vi "DAQ Main.vi"() -> ()   [LabVIEW 2017]
uses:
  Controls/RT- Queue States.ctl
  Code/TCP/TCP Engine/Controls/TCP - Driver Control State.ctl
  Code/TCP/TCP Host/Controls/Control - Testscreen.ctl
  Test cycle Execution/Control/Test Cycle Execution_States.ctl
  SubVIs/SubVI - Global.vi
  <vilib>/FPGAPlugInAG/cRIO-9034/niLvFpga_Open_cRIO-9034.vi
  <vilib>/rvi/interface/common/dynamic/niFpgaDynamicAddResources.vi
  <vilib>/Utility/error.llb/Error Cluster From Error Code.vi
  <vilib>/rvi/errors/niLvFpgaAdjustHostInterfaceError.vi
  <vilib>/Utility/file.llb/Write Delimited Spreadsheet (string).vi
  <vilib>/rvi/interface/nirviOpenFPGA/nirviOpenFPGA.xnode
  FPGA Bitfiles/TataSteel_FPGATarget_FPGA-Main_ZcEZVGyWzKA.lvbitx
  <vilib>/rvi/interface/nirviReadWriteControl/nirviReadWriteControl.xnode
  <vilib>/rvi/interface/nirviMethod/nirviMethod.xnode
  <vilib>/FPGAPlugInAG/Dynamic/niLvFpga_ReadFifo_Dynamic.vi
  <vilib>/rvi/errors/niLvFpgaMergeErrorWithErrorCode.vi
  NiFpgaLv.dll
  <vilib>/rvi/interface/Simulation/niFpgaSimulationCallBeginRW.vi
panel:
  out "SW Heartbeat":bool
  out "File Transfer":bool
  out "Datalog Interval":dbl
  out "Boolean":bool
  out "DII":bool[](array[boolean])
  out "variant":variant
  in  "Auto Trigger Data":bool
  in  "Mod1 Data":i32=2
  out "DI Data":i32[](array[numeric])
  out "Faults":bool[](array[boolean])
  out "Elapsed Time":dbl
  out "Live DI Data":u32[](array[numeric])
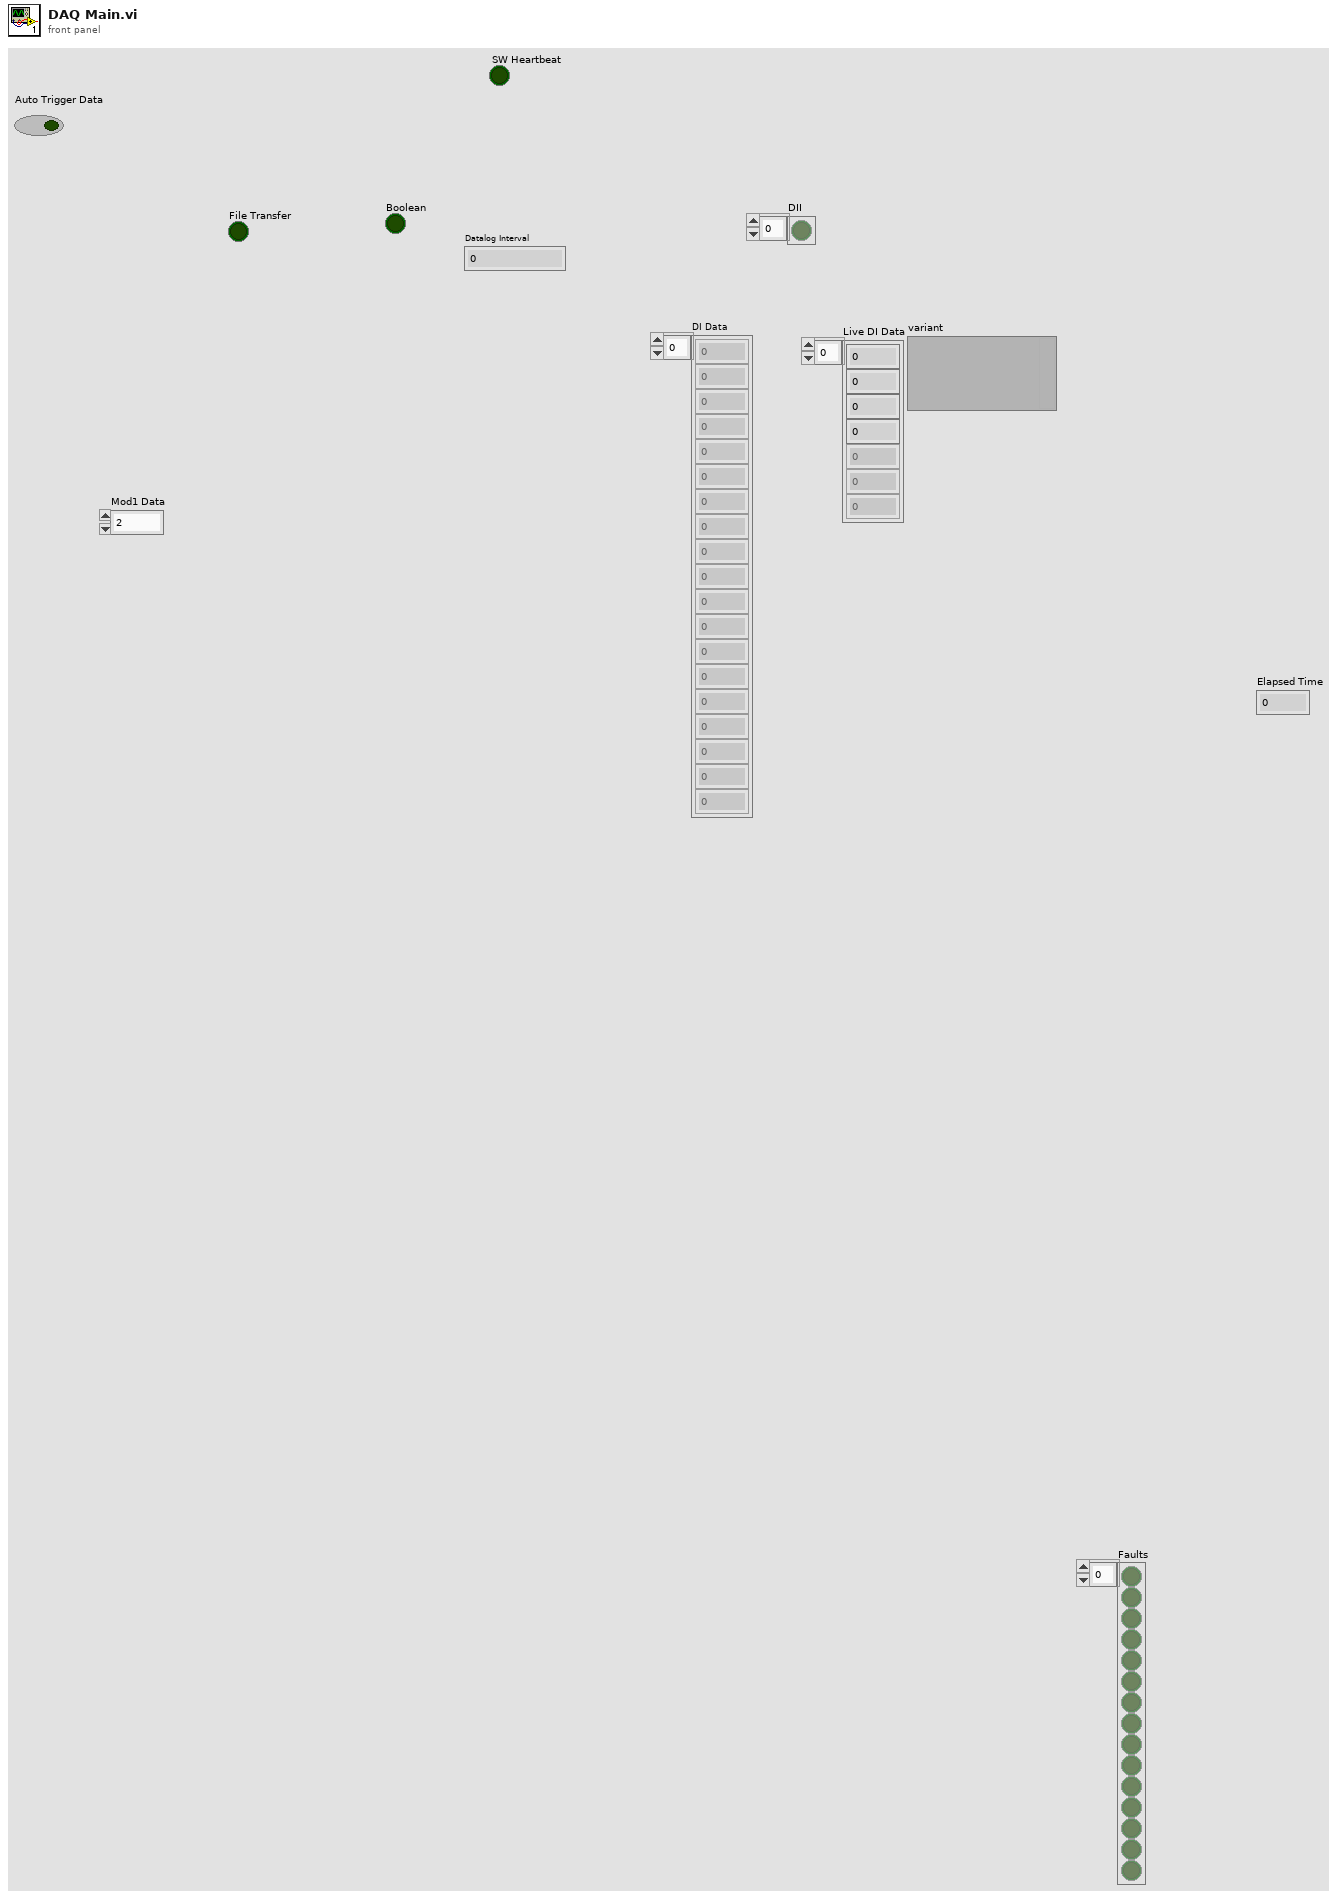
[diagram p1: front panel]
types:
  T1 = typedef "RT- Queue States.ctl" = enum16{"Initialize", "Enqueue", "Enqueue Priority", "Dequeue", "Flush", "Destroy"}
  T2 = typedef "Control - Testscreen.ctl" = enum16{"No Event", "Init", "Load Settings", "Save Setting", "Save Test Info", "Get Report", "Download Files", "Test Running", "Update Test Results", "Machine Unhealthy", "Autotest Started", "Test Aborted", "Sequence Complete", "Update Sensor Data", "Log File Available", "Machine Mode", "Aux Logging Started", "Aux File Saved", "Get PID Values", "View Report", "Exit", "Wait", "Abort", "Copy Log File", "Generate Alarm", "Send Test Details"}
  T3 = typedef "TCP - Driver Control State.ctl" = enum16{"Test Settings", "Send Test Details", "Boolean Commands", "Test Results"}
  T4 = typedef "Test Cycle Execution_States.ctl" = enum16{"Download Config Files", "Test Started", "Test Running", "Update Sensor Data", "Test Complete"}
  T5 = cluster{"Histogram Data":i16[], "Sensor Data":i16[], "File Path":path}
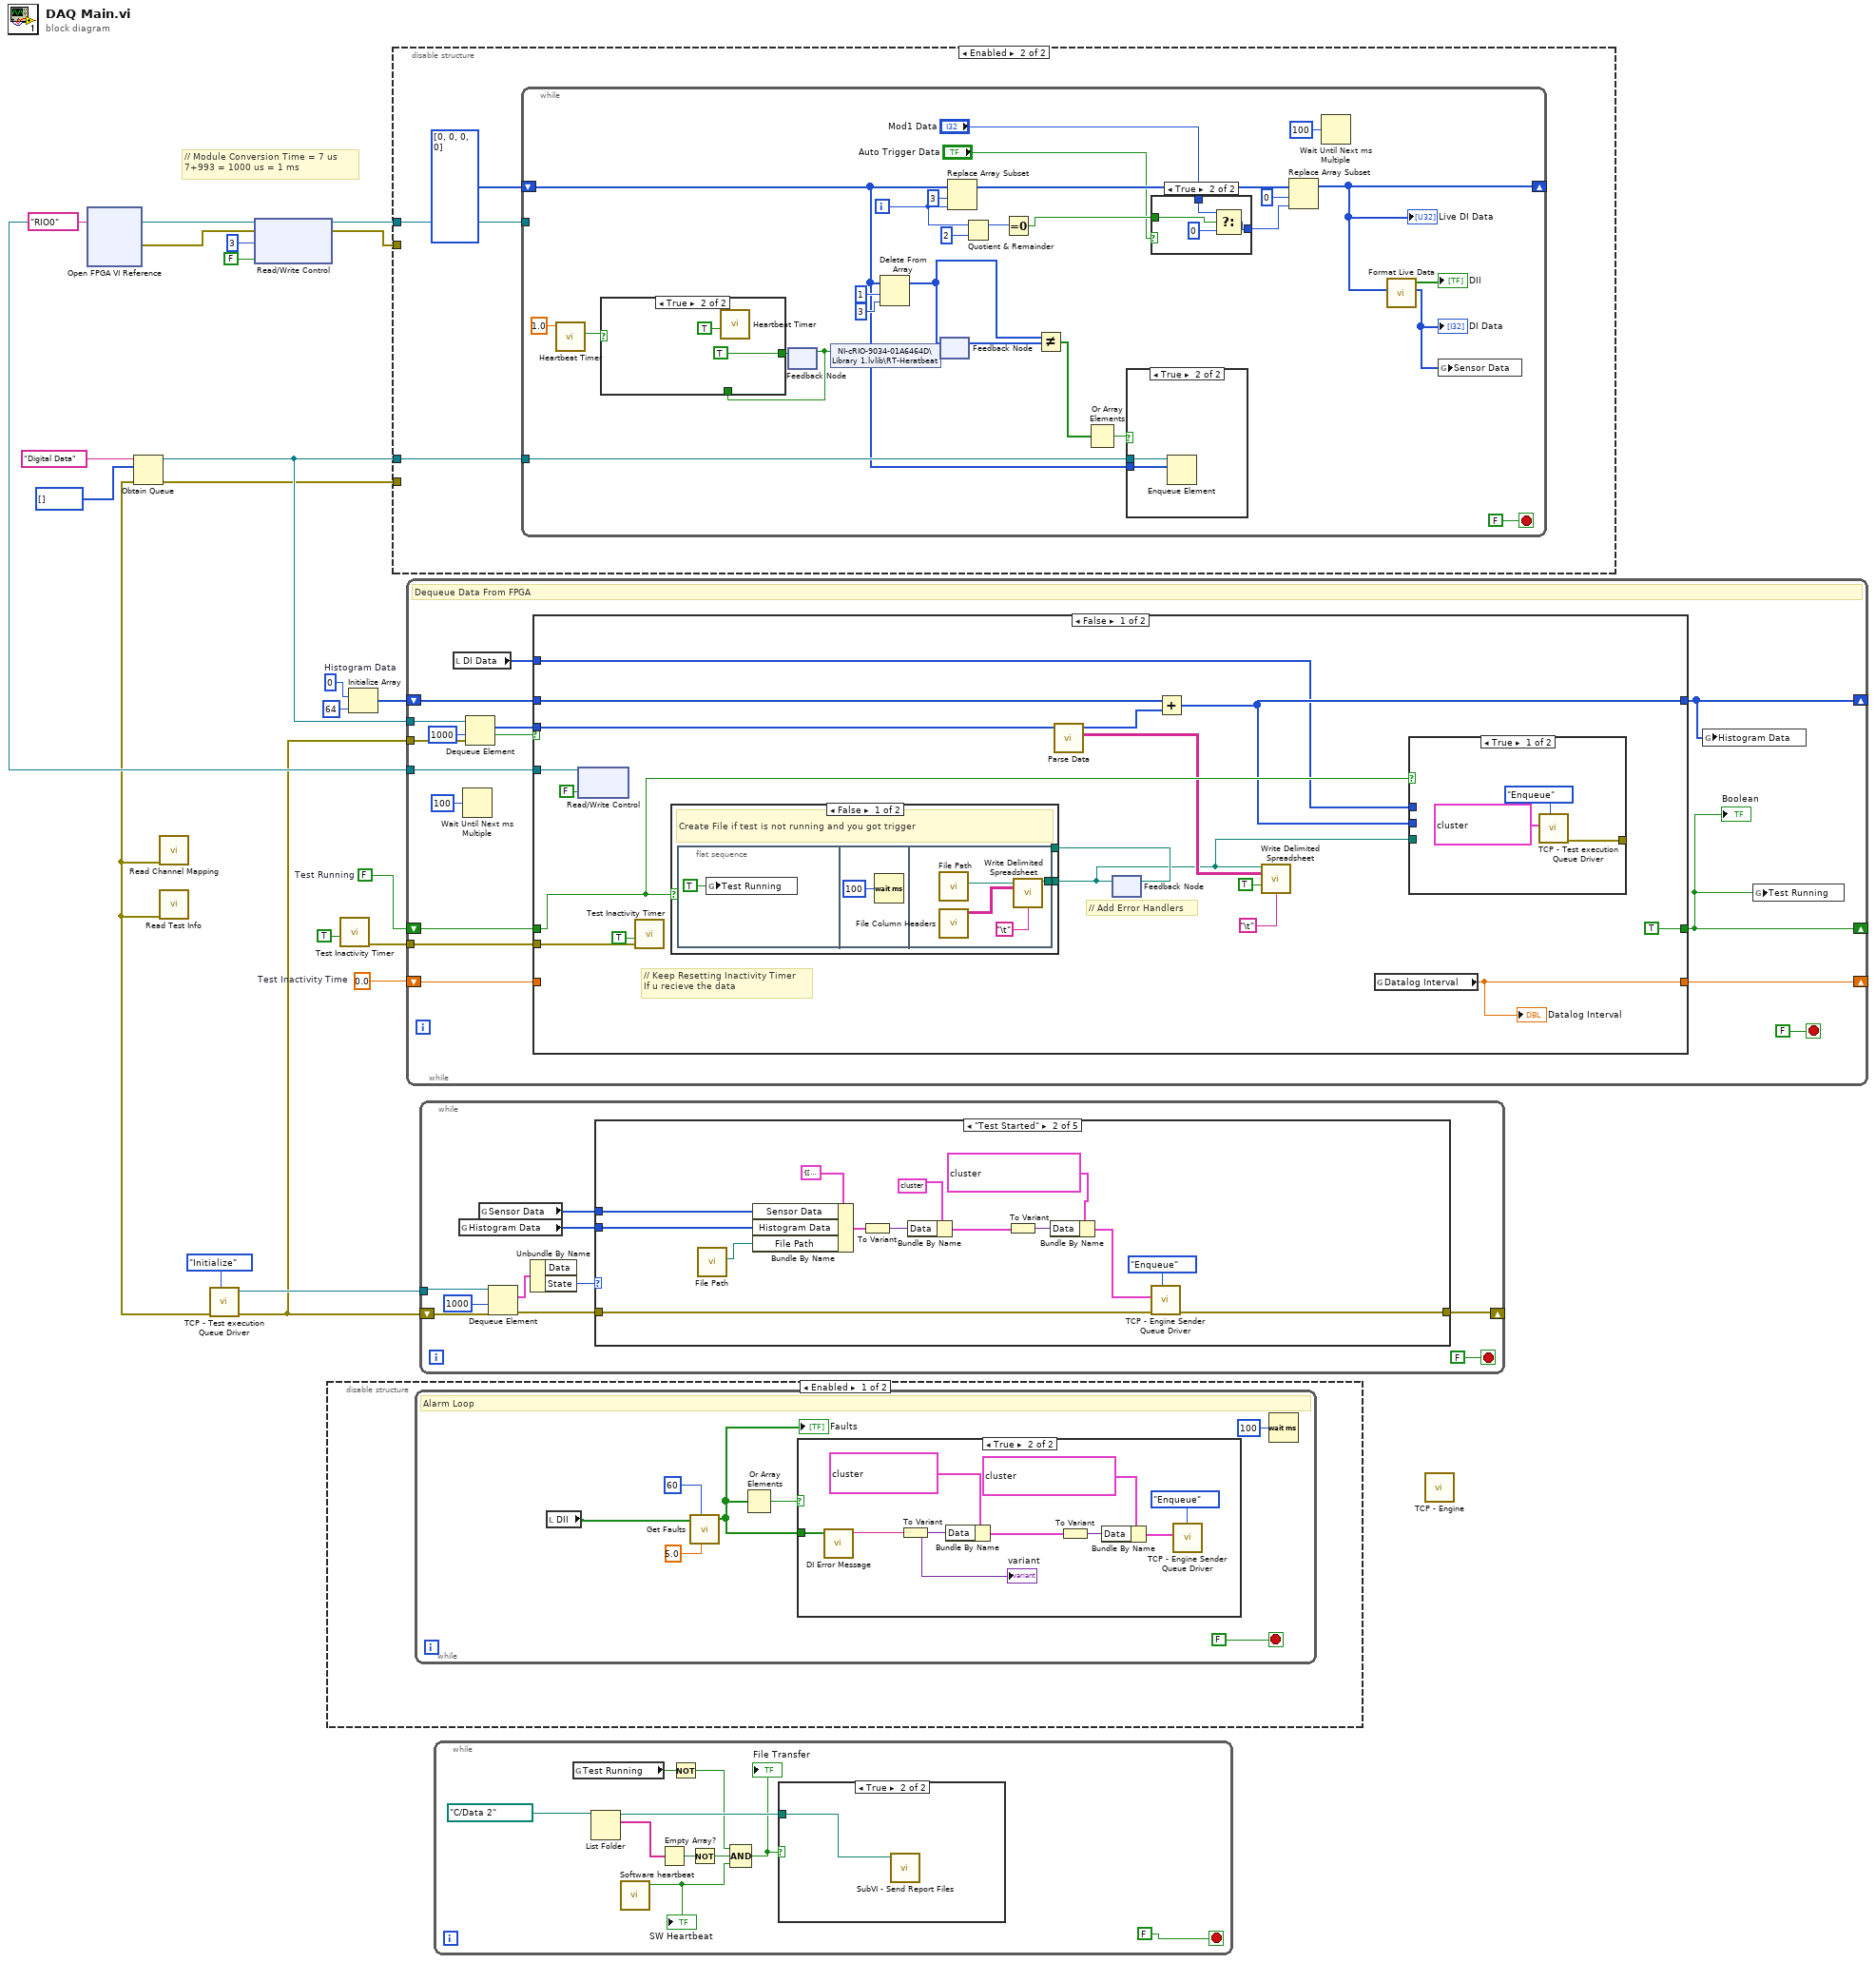
[diagram p0: block diagram]
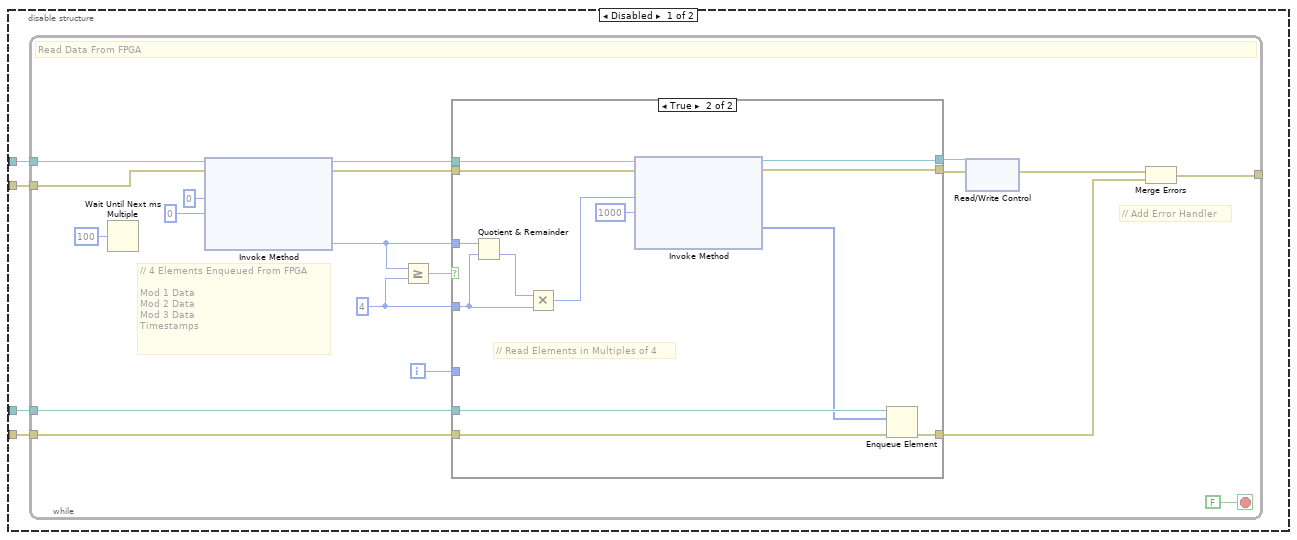
[diagram p5: hidden frame]
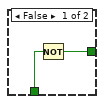
[diagram p7: hidden frame]
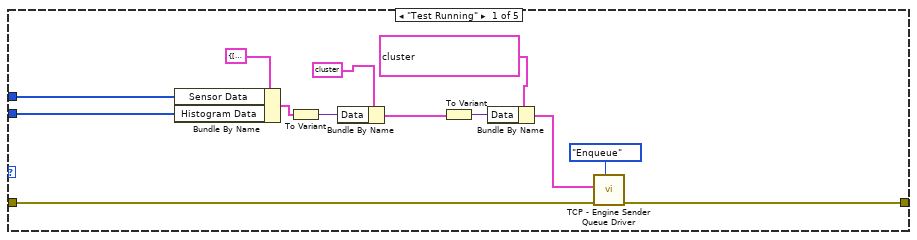
[diagram p10: hidden frame]
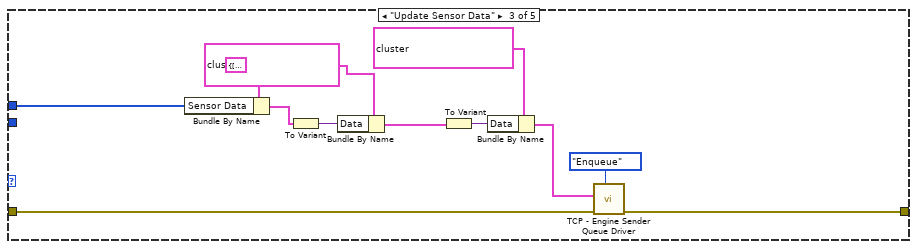
[diagram p11: hidden frame]
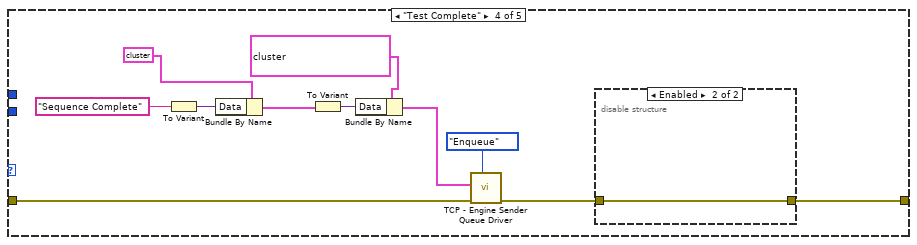
[diagram p12: hidden frame]
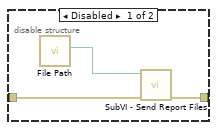
[diagram p13: hidden frame]
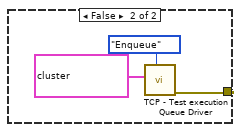
[diagram p15: hidden frame]
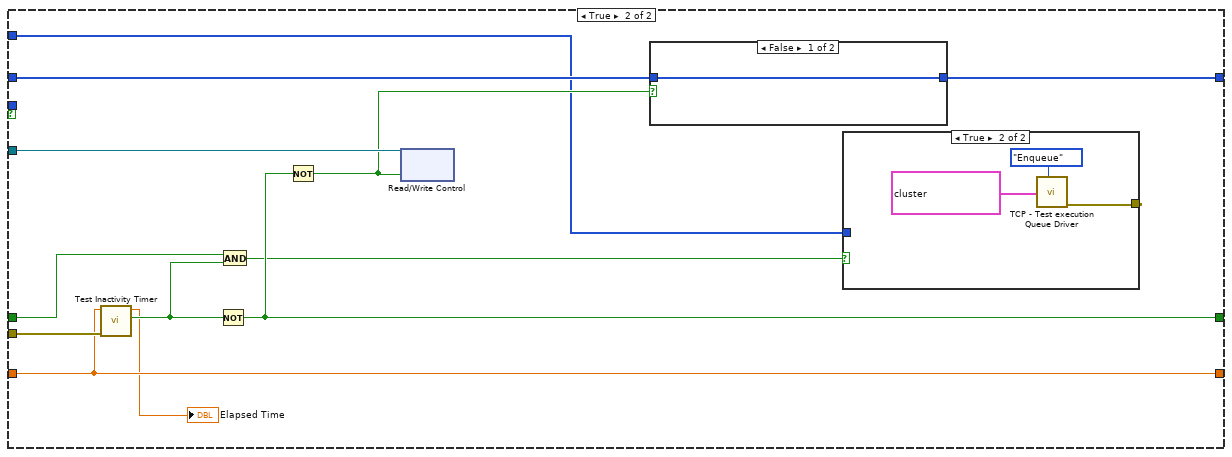
[diagram p17: hidden frame]
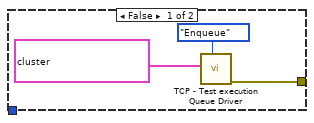
[diagram p18: hidden frame]
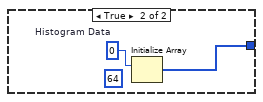
[diagram p19: hidden frame]
diagram:
  w4 = i16 0  # Histogram Data
  w15 = 0.0  # Test Inactivity Time
  w16 = FALSE  # Test Running
  # "// Module Conversion Time = 7 us\n7+993 = 1000 us = 1 ms"
  n1 = xnode "Open FPGA VI Reference"("resource name"=tag "RIO0") -> ("FPGA VI Reference Out"=w8:refnum<k20>, "error out"=w10:errorcluster)  [unwired: 1 in]
  n2 = Obtain Queue(name (unnamed)="Digital Data", element data type=u64[] [] ("Data")) -> (queue out=w19:refnum<queue>, error out=w1:errorcluster)  [unwired: 3 in, 1 out]
  n3 = call "Read Channel Mapping.vi"("error in (no error)"=w1) -> ()  [unwired: 11 in]
  n4 = call "Read Test Info.vi"("error in (no error)"=w1) -> ()  [unwired: 11 in]
  n5 = call "TCP - Test execution Queue Driver.vi"("Cases"=RT-_Queue_States."Initialize", "error in (no error)"=w1) -> ("error out"=w5:errorcluster, "queue out"=w6:refnum<queue>)  [unwired: 7 in, 1 out]
  n6 = xnode "Read/Write Control"("FPGA VI Reference In"=w8, "error in"=w10, "Wait(uSec)"=u32 3, "Manual Log"=FALSE) -> ("FPGA VI Reference Out"=w12:refnum<k20>, "error out"=w9:errorcluster)
  n7 = disable-structure shown="Enabled" {
    frame Enabled {
      n8 = while {
        stop <- FALSE ("stop") stop-if-true
        # "Alarm Loop"
        n9 = local read "DII"() -> (w22:bool[])
        n10 = call "Get Faults.vi"("Timer(Sec)"=5.0, "No of Inputs"=60, "Inputs"=w22) -> ("Faults"=w23:bool[])  [unwired: 8 in]
        "Faults" <- w23
        n11 = Or Array Elements(Boolean array=w23) -> (logical OR=w24:bool)
        n12 = case shown="True" w24 {
          tunnel: w23 -> [_ w33]
          frame False {
          }
          frame True {
            n13 = call "DI Error Message.vi"("Faults"=w33) -> ("Error Message"=w29:string)  [unwired: 10 in]
            n14 = To Variant(anything=w29) -> (Variant=w36:variant)
            "variant" <- w36
            n15 = Bundle By Name(cluster=cluster{"Data":variant, "Enum":T2} {"Data"=variant, "Enum"=enum."Generate Alarm"} ("Element In"), "Data"=w36) -> (w32:cluster{"Data":variant, "Enum":T2})
            n16 = To Variant(anything=w32) -> (Variant=w37:variant)
            n17 = Bundle By Name(cluster=cluster{"Data":variant, "State":T3} {"Data"=variant, "State"=enum."Boolean Commands"} ("Element In"), "Data"=w37) -> (w35:cluster{"Data":variant, "State":T3})
            n18 = call "TCP - Engine Sender Queue Driver.vi"("Cases"=RT-_Queue_States."Enqueue", "Element In"=w35) -> ()  [unwired: 7 in, 3 out]
          }
        }
        n19 = Wait (ms)(milliseconds to wait=u32 100) -> ()  [unwired: 1 out]
      }
    }
    frame Disabled {
    }
  }
  n20 = call "Test Inactivity Timer.vi"("Reset"=TRUE) -> ("error out"=w17:errorcluster)  [unwired: 8 in, 2 out]
  n21 = Initialize Array(w4, 64 ("dimension size")) -> (w3:i16[])
  n22 = disable-structure shown="Enabled" {
    disable-tunnel: w19 -> [w41 w78]
    disable-tunnel: w12 -> [w40 w79]
    disable-tunnel: w9 -> [w39 _]
    disable-tunnel: w1 -> [w38 _]
    frame Disabled {
      n23 = while {
        tunnel: w40 -> [w45]
        tunnel: w39 -> [w55]
        tunnel: w41 -> [w52]
        tunnel: w38 -> [w51]
        tunnel: [w49] -> _
        i -> [w46]
        stop <- FALSE stop-if-true
        w57 = u32 4 ("y")
        # "// Add Error Handler"
        # "// 4 Elements Enqueued From FPGA\n\nMod 1 Data\nMod 2 Data\nMod 3 Data\nTimestamps"
        # "Read Data From FPGA"
        n24 = Wait Until Next ms Multiple(millisecond multiple=u32 100) -> ()  [unwired: 1 out]
        n25 = xnode "Invoke Method"("FPGA VI Reference In"=w45, "error in"=w55, "Number of Elements"=u32 0, "Timeout (ms)"=0) -> ("FPGA VI Reference Out"=w54:refnum<k20>, "error out"=w53:errorcluster, "Elements Remaining"=w58:u32)  [unwired: 1 out]
        n26 = Greater Or Equal?(x=w58, y=w57) -> (x >= y?=w56:bool)
        n27 = case shown="True" w56 {
          tunnel: w58 -> [_ w76]
          tunnel: w57 -> [_ w74]
          tunnel: w54 -> [w61 w73]
          tunnel: w53 -> [w63 w72]
          tunnel: w52 -> [_ w69]
          tunnel: w51 -> [w62 w68]
          tunnel: [w63 w66] -> w43
          tunnel: [w62 w65] -> w50
          tunnel: w46 -> [_ _]
          tunnel: [w61 w64] -> w44
          frame False {
          }
          frame True {
            # "// Read Elements in Multiples of 4"
            n28 = Quotient & Remainder(x=w76, y=w74) -> (floor(x/y)=w75:u32)  [unwired: 1 out]
            n29 = Multiply(x=w75, y=w74) -> (x*y=w71:u32)
            n30 = xnode "Invoke Method"("FPGA VI Reference In"=w73, "error in"=w72, "Number of Elements"=w71, "Timeout (ms)"=1000) -> ("FPGA VI Reference Out"=w64:refnum<k20>, "error out"=w66:errorcluster, "Data"=w67:u64[])  [unwired: 1 out]
            n31 = Enqueue Element(queue=w69, element=w67, error in (no error)=w68) -> (error out=w65:errorcluster)  [unwired: 1 in, 2 out]
          }
        }
        n32 = xnode "Read/Write Control"("FPGA VI Reference In"=w44, "error in"=w43) -> ("error out"=w42:errorcluster)  [unwired: 2 out]
        n33 = Merge Errors(w42, w50) -> (w49:errorcluster)
      }
    }
    frame Enabled {
      n34 = while {
        tunnel: w79 -> [_]
        tunnel: w78 -> [w106]
        shift-right: [w92] -> _
        shift-left: u32[] [0, 0, 0, 0] ("Simulation") -> [w89]
        i -> [w98]
        stop <- FALSE stop-if-true
        n35 = call "Heartbeat Timer.vi"("Target Time"=1.0) -> ("Time Elapsed"=w83:bool)  [unwired: 8 in, 2 out]
        n36 = feedback #1() -> (w80:bool)  [unwired: 1 in]
        n37 = case shown="True" w83 {
          tunnel: [w107 TRUE] -> w81
          tunnel: w80 -> [w108 _]
          frame False {
            n38 = Not(x=w108) -> (.not. x?=w107:bool)
          }
          frame True {
            n39 = call "Heartbeat Timer.vi"("Reset"=TRUE) -> ()  [unwired: 8 in, 3 out]
          }
        }
        n40 = feedback-in #1(w81) -> ()
        n41 = shared-variable "NI-cRIO-9034-01A6464D\\Library 1.lvlib\\RT-Heratbeat"(w80) -> ()  [unwired: 1 in, 1 out]
        n42 = Delete From Array(array=w89, length=1, index=3) -> (array with subset deleted=w88:u32[])  [unwired: 1 out]
        n43 = feedback-in #2(w88) -> ()
        n44 = feedback #2() -> (w104:u32[])  [unwired: 1 in]
        n45 = Replace Array Subset(array=w89, new element=w98, index=3) -> (w99:u32[])
        n46 = Quotient & Remainder(x=w98, y=2) -> (x-y*floor(x/y)=w96:i32)  [unwired: 1 out]
        n47 = Equal To 0?(x=w96) -> (x = 0?=w87:bool)
        n48 = Not Equal?(x=w88, y=w104) -> (x != y?=w103:bool[])
        n49 = Or Array Elements(Boolean array=w103) -> (logical OR=w102:bool)
        n50 = case shown="True" w102 {
          tunnel: w106 -> [_ w117]
          tunnel: w89 -> [_ w116]
          frame False {
          }
          frame True {
            n51 = Enqueue Element(queue=w117, element=w116) -> ()  [unwired: 2 in, 3 out]
          }
        }
        n52 = case shown="True" "Auto Trigger Data" {
          tunnel: "Mod1 Data" -> [w111 w115]
          tunnel: [w111 w113] -> w94
          tunnel: w87 -> [_ w112]
          frame False {
          }
          frame True {
            n53 = Select(t=w115, s=w112, f=0) -> (s? t:f=w113:i32)
          }
        }
        n54 = Replace Array Subset(array=w99, new element=w94, index=0) -> (w92:u32[])
        "Live DI Data" <- w92
        n55 = Wait Until Next ms Multiple(millisecond multiple=u32 100) -> ()  [unwired: 1 out]
        n56 = call "Format Live Data.vi"("Live DI Data"=w92) -> ("Array"=w105:i16[], "DII"=→"DII":bool[])  [unwired: 9 in]
        "DI Data" <- w105
        n57 = global write "SubVI - Global.vi" "Sensor Data"(w105) -> ()
      }
    }
  }
  n58 = while {
    tunnel: w19 -> [w133]
    tunnel: w5 -> [w132]
    tunnel: w17 -> [w127]
    shift-right: [w118] -> _
    shift-left: w16 -> [w126]
    shift-right: [w124] -> _
    shift-left: w15 -> [w125]
    tunnel: w8 -> [w122]
    shift-right: [w119] -> _
    shift-left: w3 -> [w121]
    stop <- FALSE stop-if-true
    # "Dequeue Data From FPGA"
    n59 = local read "DI Data"() -> (w120:i32[])
    n60 = Wait Until Next ms Multiple(millisecond multiple=u32 100) -> ()  [unwired: 1 out]
    n61 = Dequeue Element(queue=w133, timeout in ms (-1)=1000, error in (no error)=w132) -> (element=w131:u64[], timed out?=w128:bool)  [unwired: 2 out]
    n62 = case shown="False" w128 {
      tunnel: w131 -> [w150 _]
      tunnel: w127 -> [w148 w176]
      tunnel: w126 -> [w144 w167]
      tunnel: [TRUE w173] -> w118
      tunnel: w125 -> [_ w175]
      tunnel: [w135 w175] -> w124
      tunnel: w122 -> [w141 w174]
      tunnel: w121 -> [w143 w171]
      tunnel: [w142 w170] -> w119
      tunnel: w120 -> [w136 w165]
      frame False {
        # "// Add Error Handlers"
        # "// Keep Resetting Inactivity Timer\nIf u recieve the data"
        n63 = xnode "Read/Write Control"("FPGA VI Reference In"=w141, "Reset"=FALSE) -> ()  [unwired: 1 in, 2 out]
        n64 = call "Test Inactivity Timer.vi"("error in (no error)"=w148, "Reset"=TRUE) -> ()  [unwired: 7 in, 3 out]
        n65 = call "Parse Data.vi"("Data In"=w150) -> ("Values to Log"=w139:string[][], "Histogram Data"=w138:i16[])  [unwired: 9 in]
        n66 = feedback #3() -> (w145:path)  [unwired: 1 in]
        n67 = case shown="False" w144 {
          tunnel: [w157 w164] -> w137
          tunnel: w145 -> [_ w164]
          frame False {
            # "Create File if test is not running and you got trigger"
            n68 = flat-sequence {
              tunnel: [w162] -> w157
              frame #0 {
                n69 = global write "SubVI - Global.vi" "Test Running"(TRUE ("Test Running")) -> ()
              }
              frame #1 {
                n70 = Wait (ms)(milliseconds to wait=u32 100) -> ()  [unwired: 1 out]
              }
              frame #2 {
                n71 = call "File Path.vi"() -> ("File Path"=w161:path)  [unwired: 11 in]
                n72 = call "File Column Headers.vi"() -> ("Column Header"=w163:string[][])  [unwired: 11 in]
                n73 = call-poly <vilib>:"Write Delimited Spreadsheet.vi"("file path (dialog if empty)"=w161, "2D data"=w163, "delimiter (\\t)"="\t") -> ("new file path (Not A Path if cancelled)"=w162:path)  [unwired: 11 in, 1 out]
              }
            }
          }
          frame True {
          }
        }
        n74 = feedback-in #3(w137) -> ()
        n75 = Add(x=w143, y=w138) -> (x+y=w142:i16[])
        n76 = call-poly <vilib>:"Write Delimited Spreadsheet.vi"("file path (dialog if empty)"=w137, "2D data"=w139, "append to file? (new file:F)"=TRUE, "delimiter (\\t)"="\t") -> ()  [unwired: 10 in, 2 out]
        n77 = global read "SubVI - Global.vi" "Datalog Interval"() -> (w135:dbl)
        "Datalog Interval" <- w135
        n78 = case shown="True" w144 {
          tunnel: w136 -> [_ _]
          tunnel: w142 -> [_ _]
          tunnel: [w152 w155] -> _
          tunnel: w137 -> [_ _]
          frame True {
            n79 = call "TCP - Test execution Queue Driver.vi"("Cases"=RT-_Queue_States."Enqueue", "Element In"=cluster{"Data":variant, "State":T4} {"Data"=variant, "State"=enum."Test Running"}) -> ("error out"=w152:errorcluster)  [unwired: 7 in, 2 out]
          }
          frame False {
            n80 = call "TCP - Test execution Queue Driver.vi"("Cases"=RT-_Queue_States."Enqueue", "Element In"=cluster{"Data":variant, "State":T4} {"Data"=variant, "State"=enum."Test Started"}) -> ("error out"=w155:errorcluster)  [unwired: 7 in, 2 out]
          }
        }
      }
      frame True {
        n81 = call "Test Inactivity Timer.vi"("error in (no error)"=w176, "Target Time"=w175) -> ("Time Elapsed"=w169:bool, "Elapsed Time"=→"Elapsed Time":dbl)  [unwired: 7 in, 1 out]
        n82 = Not(x=w169) -> (.not. x?=w173:bool)
        n83 = And(x=w167, y=w169) -> (x .and. y?=w168:bool)
        n84 = Not(x=w173) -> (.not. x?=w172:bool)
        n85 = xnode "Read/Write Control"("FPGA VI Reference In"=w174, "Reset"=w172) -> ()  [unwired: 1 in, 2 out]
        n86 = case shown="False" w172 {
          tunnel: w171 -> [w183 _]
          tunnel: [w183 w184] -> w170
          frame False {
          }
          frame True {
            (unwired) 64 ("dimension size")
            w185 = i16 0  # Histogram Data
            n87 = Initialize Array(w185) -> (w184:i16[])  [unwired: 1 in]
          }
        }
        n88 = case shown="True" w168 {
          tunnel: w165 -> [_ _]
          tunnel: [w179 w182] -> _
          frame False {
            n89 = call "TCP - Test execution Queue Driver.vi"("Cases"=RT-_Queue_States."Enqueue", "Element In"=cluster{"Data":variant, "State":T4} {"Data"=variant, "State"=enum."Update Sensor Data"}) -> ("error out"=w179:errorcluster)  [unwired: 7 in, 2 out]
          }
          frame True {
            n90 = call "TCP - Test execution Queue Driver.vi"("Cases"=RT-_Queue_States."Enqueue", "Element In"=cluster{"Data":variant, "State":T4} {"Data"=variant, "State"=enum."Test Complete"}) -> ("error out"=w182:errorcluster)  [unwired: 7 in, 2 out]
          }
        }
      }
    }
    "Boolean" <- w118
    n91 = global write "SubVI - Global.vi" "Histogram Data"(w119) -> ()
    n92 = global write "SubVI - Global.vi" "Test Running"(w118) -> ()
  }
  n93 = while {
    shift-right: [w192] -> _
    shift-left: w5 -> [w193]
    tunnel: w6 -> [w194]
    stop <- FALSE stop-if-true
    n94 = global read "SubVI - Global.vi" "Histogram Data"() -> (w188:i32[])
    n95 = global read "SubVI - Global.vi" "Sensor Data"() -> (w187:i32[])
    n96 = Dequeue Element(queue=w194, timeout in ms (-1)=1000, error in (no error)=w193) -> (element=w190:cluster{"Data":variant, "State":T4}, error out=w191:errorcluster)  [unwired: 2 out]
    n97 = Unbundle By Name(w190) -> ("State"=w189:T4)  [unwired: 1 out]
    n98 = case shown="\"Test Started\"" w189 {
      tunnel: [w199 w213 w226 w238 w250] -> w192
      tunnel: w191 -> [w200 w214 w227 w241 w250]
      tunnel: w188 -> [w202 w216 _ _ _]
      tunnel: w187 -> [w201 w215 w228 _ _]
      frame "Test Running" {
        n99 = Bundle By Name(cluster=T5 {"Histogram Data"=[], "Sensor Data"=[], "File Path"=path ""}, "Sensor Data"=w201, "Histogram Data"=w202) -> (w208:T5)
        n100 = To Variant(anything=w208) -> (Variant=w206:variant)
        n101 = Bundle By Name(cluster=cluster{"Data":variant, "Enum":T2} {"Data"=variant, "Enum"=enum."Test Running"} ("Element In"), "Data"=w206) -> (w197:cluster{"Data":variant, "Enum":T2})
        n102 = To Variant(anything=w197) -> (Variant=w207:variant)
        n103 = Bundle By Name(cluster=cluster{"Data":variant, "State":T3} {"Data"=variant, "State"=enum."Boolean Commands"} ("Element In"), "Data"=w207) -> (w205:cluster{"Data":variant, "State":T3})
        n104 = call "TCP - Engine Sender Queue Driver.vi"("Cases"=RT-_Queue_States."Enqueue", "error in (no error)"=w200, "Element In"=w205) -> ("error out"=w199:errorcluster)  [unwired: 6 in, 2 out]
      }
      frame "Test Started" {
        n105 = call "File Path.vi"() -> ("File Path"=w209:path)  [unwired: 11 in]
        n106 = Bundle By Name(cluster=T5 {"Histogram Data"=[], "Sensor Data"=[], "File Path"=path ""}, "Sensor Data"=w215, "Histogram Data"=w216, "File Path"=w209) -> (w222:T5)
        n107 = To Variant(anything=w222) -> (Variant=w220:variant)
        n108 = Bundle By Name(cluster=cluster{"Data":variant, "Enum":T2} {"Data"=variant, "Enum"=enum."Autotest Started"} ("Element In"), "Data"=w220) -> (w211:cluster{"Data":variant, "Enum":T2})
        n109 = To Variant(anything=w211) -> (Variant=w221:variant)
        n110 = Bundle By Name(cluster=cluster{"Data":variant, "State":T3} {"Data"=variant, "State"=enum."Boolean Commands"} ("Element In"), "Data"=w221) -> (w219:cluster{"Data":variant, "State":T3})
        n111 = call "TCP - Engine Sender Queue Driver.vi"("Cases"=RT-_Queue_States."Enqueue", "error in (no error)"=w214, "Element In"=w219) -> ("error out"=w213:errorcluster)  [unwired: 6 in, 2 out]
      }
      frame "Update Sensor Data" {
        n112 = Bundle By Name(cluster=T5 {"Histogram Data"=[], "Sensor Data"=[], "File Path"=path ""}, "Sensor Data"=w228) -> (w234:T5)
        n113 = To Variant(anything=w234) -> (Variant=w232:variant)
        n114 = Bundle By Name(cluster=cluster{"Data":variant, "Enum":T2} {"Data"=variant, "Enum"=enum."Update Sensor Data"} ("Element In"), "Data"=w232) -> (w224:cluster{"Data":variant, "Enum":T2})
        n115 = To Variant(anything=w224) -> (Variant=w233:variant)
        n116 = Bundle By Name(cluster=cluster{"Data":variant, "State":T3} {"Data"=variant, "State"=enum."Boolean Commands"} ("Element In"), "Data"=w233) -> (w231:cluster{"Data":variant, "State":T3})
        n117 = call "TCP - Engine Sender Queue Driver.vi"("Cases"=RT-_Queue_States."Enqueue", "error in (no error)"=w227, "Element In"=w231) -> ("error out"=w226:errorcluster)  [unwired: 6 in, 2 out]
      }
      frame "Test Complete" {
        n118 = To Variant(anything="Sequence Complete") -> (Variant=w244:variant)
        n119 = Bundle By Name(cluster=cluster{"Data":variant, "Enum":T2} {"Data"=variant, "Enum"=enum."Sequence Complete"} ("Element In"), "Data"=w244) -> (w236:cluster{"Data":variant, "Enum":T2})
        n120 = To Variant(anything=w236) -> (Variant=w245:variant)
        n121 = Bundle By Name(cluster=cluster{"Data":variant, "State":T3} {"Data"=variant, "State"=enum."Boolean Commands"} ("Element In"), "Data"=w245) -> (w243:cluster{"Data":variant, "State":T3})
        n122 = call "TCP - Engine Sender Queue Driver.vi"("Cases"=RT-_Queue_States."Enqueue", "error in (no error)"=w241, "Element In"=w243) -> ("error out"=w239:errorcluster)  [unwired: 6 in, 2 out]
        n123 = disable-structure shown="Enabled" {
          disable-tunnel: w239 -> [w247 w249]
          disable-tunnel: [w246 w249] -> w238
          frame Disabled {
            n124 = call "File Path.vi"() -> ("File Path"=w248:path)  [unwired: 11 in]
            n125 = call "SubVI - Send Report Files.vi"("error in (no error)"=w247, "file path (use dialog)"=w248) -> ("error out"=w246:errorcluster)  [unwired: 9 in]
          }
          frame Enabled {
          }
        }
      }
      frame "Download Config Files" {
      }
    }
  }
  n126 = while {
    stop <- FALSE ("stop") stop-if-true
    n127 = global read "SubVI - Global.vi" "Test Running"() -> (w254:bool)
    n128 = List Folder(path=path "C:/Data 2") -> (path out=w259:path, filenames=w258:string[])  [unwired: 3 in, 2 out]
    n129 = call "Software heartbeat.vi"() -> ("SW Heartbeat"=w251:bool)  [unwired: 11 in]
    "SW Heartbeat" <- w251
    n130 = Empty Array?(array=w258) -> (empty?=w257:bool)
    n131 = Not(x=w254) -> (.not. x?=w252:bool)
    n132 = Not(x=w257) -> (.not. x?=w253:bool)
    n133 = Compound Arithmetic op=AND(w252, w253, w251) -> (w255:bool)
    "File Transfer" <- w255
    n134 = case shown="True" w255 {
      tunnel: w259 -> [_ w261]
      frame False {
      }
      frame True {
        n135 = call "SubVI - Send Report Files.vi"("file path (use dialog)"=w261) -> ()  [unwired: 10 in, 1 out]
      }
    }
  }
  n136 = call "TCP - Engine.vi"() -> ()  [unwired: 12 in]
